vi "SetGains.vi"(0 "Interface in":T2, 5 "Gains":T1, 11 "error in":errorcluster) -> (4 "Interface out":T2, 15 "error out":errorcluster)   [LabVIEW 2017, in "AFE_interface.lvlib"]
uses:
  AFE_interface.lvlib
  InterfaceRef.ctl
  <instrlib>/_niInstr/Instruction Framework/v1/Host/Instruction Target/niInstr Instruction Target v1 Host.lvclass
  <instrlib>/_niInstr/Instruction Framework/v1/Host/Instruction Framework Context/niInstr Instruction Framework Context v1 Host.lvclass
  AFE/Gains.ctl
  AFE/ActiveFrontEnd.lvlib
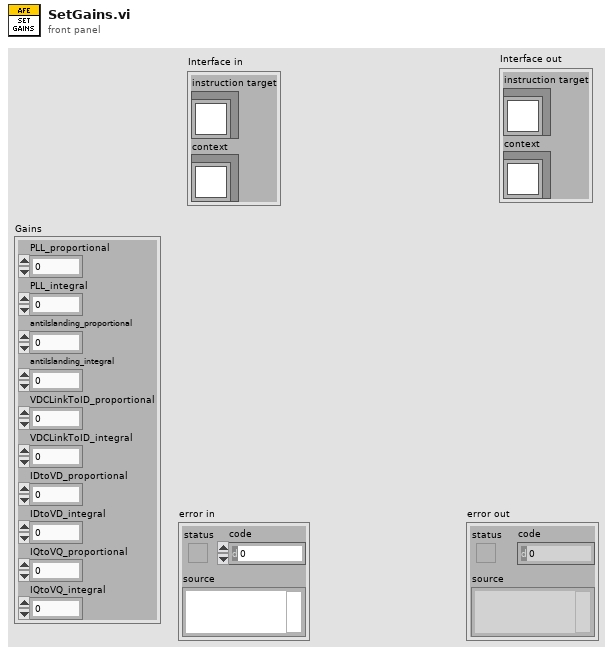
[diagram p1: front panel]
types:
  T1 = typedef "ActiveFrontEnd.lvlib/Gains.ctl" = cluster{"PLL_proportional":sgl, "PLL_integral":sgl, "antiIslanding_proportional":sgl, "antiIslanding_integral":sgl, "VDCLinkToID_proportional":sgl, "VDCLinkToID_integral":sgl, "IDtoVD_proportional":sgl, "IDtoVD_integral":sgl, "IQtoVQ_proportional":sgl, "IQtoVQ_integral":sgl}
  T2 = typedef "AFE_interface.lvlib/InterfaceRef.ctl" = cluster{"instruction target":refnum<class "niInstr Instruction Target v1 Host.lvclass">, "context":refnum<class "niInstr Instruction Framework Context v1 Host.lvclass">}
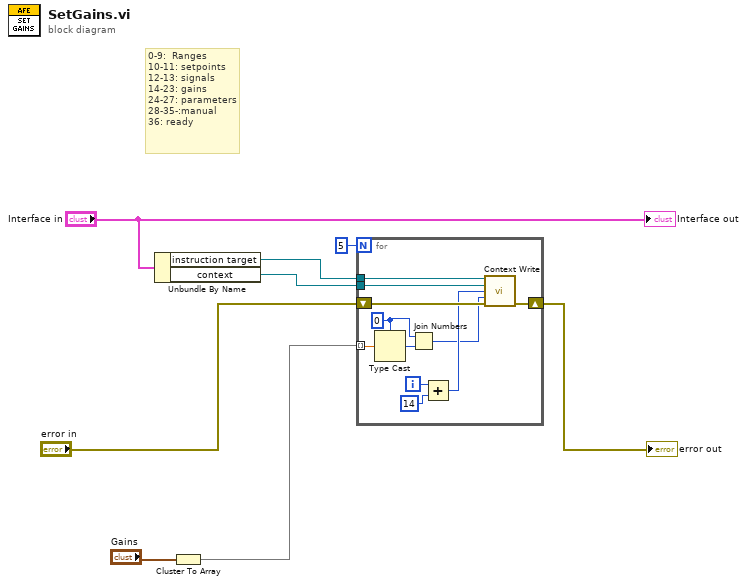
[diagram p0: block diagram]
diagram:
  # "0-9:  Ranges\n10-11: setpoints\n12-13: signals\n14-23: gains\n24-27: parameters\n28-35-:manual\n36: ready"
  n1 = Unbundle By Name("Interface in") -> ("instruction target"=w7:refnum<class "niInstr Instruction Target v1 Host.lvclass">, "context"=w6:refnum<class "niInstr Instruction Framework Context v1 Host.lvclass">)
  n2 = Cluster To Array(cluster="Gains") -> (array=w2:sgl[])
  n3 = for {
    N: 5 -> [_]
    tunnel: w7 -> [w19]
    tunnel: w6 -> [w18]
    shift-right: [w16] -> w4
    shift-left: "error in" -> [w17]
    tunnel: w2 -> [w12] mode=indexing
    i -> [w13]
    w11 = u32 0
    n4 = Type Cast(type=w11, x=w12) -> (*(type *) &x=w10:u32)
    n5 = Join Numbers(hi=w11, lo=w10) -> ((hi.lo)=w9:u64)
    n6 = Add(x=w13, y=14) -> (x+y=w14:i32)
    n7 = call <instrlib>:"Context Write.vi"("instruction target in"=w19, "context in"=w18, "address"=w14, "data"=w9, "error in"=w17) -> ("error out"=w16:errorcluster)  [unwired: 8 in, 2 out]
  }
  "error out" <- w4
  "Interface out" <- "Interface in"
